vi "Auto Generate Reports.vi"(9 "Report Parameters":T2(array[cluster])=[{"output file suffix"="TSM_SSC", "dir filter"="^\\b(?:(?!SSC|Single SSC)\\w)+\\b"}, {"output file suffix"="SSC", "dir filter"="^SSC|^Single SSC "}], 10 "output file path":path=path "docs", 11 "search dir":path=path "C:/ADIBitbucket/nists19.0_templateproject/Code Modules/Common/Instrument Control") -> (0 "error out":errorcluster={"status"=TRUE, "code"=118, "source"="Invoke Node in VI Documenation MD Report Gen.lvlib:Format VI Information.vi:2500001->VI Documenation MD Report Gen.lvlib:Generate Documentation from VIs.vi->VI Documenation MD Report Gen.lvlib:Auto Generate Reports.vi\n<APPEND>\nMethod Name: <b>Print:VI To HTML</b>"}, 1 "Report Text":string[](array[string]), 3 "Report Files":path[](array[path])=[path "C:/Users/marobert/Desktop/STSDevToolsDocProj/LV Documenation to MD/VI Documenation MD Report Gen/docs/Waveform Acquisition_TSM_SSC.md", path "C:/Users/marobert/Desktop/STSDevToolsDocProj/LV Documenation to MD/VI Documenation MD Report Gen/docs/Waveform Acquisition_SSC.md"])   [LabVIEW 2019, in "MD Generator.lvlib"]
uses:
  MD Generator.lvlib
  subVIs/Filter.ctl
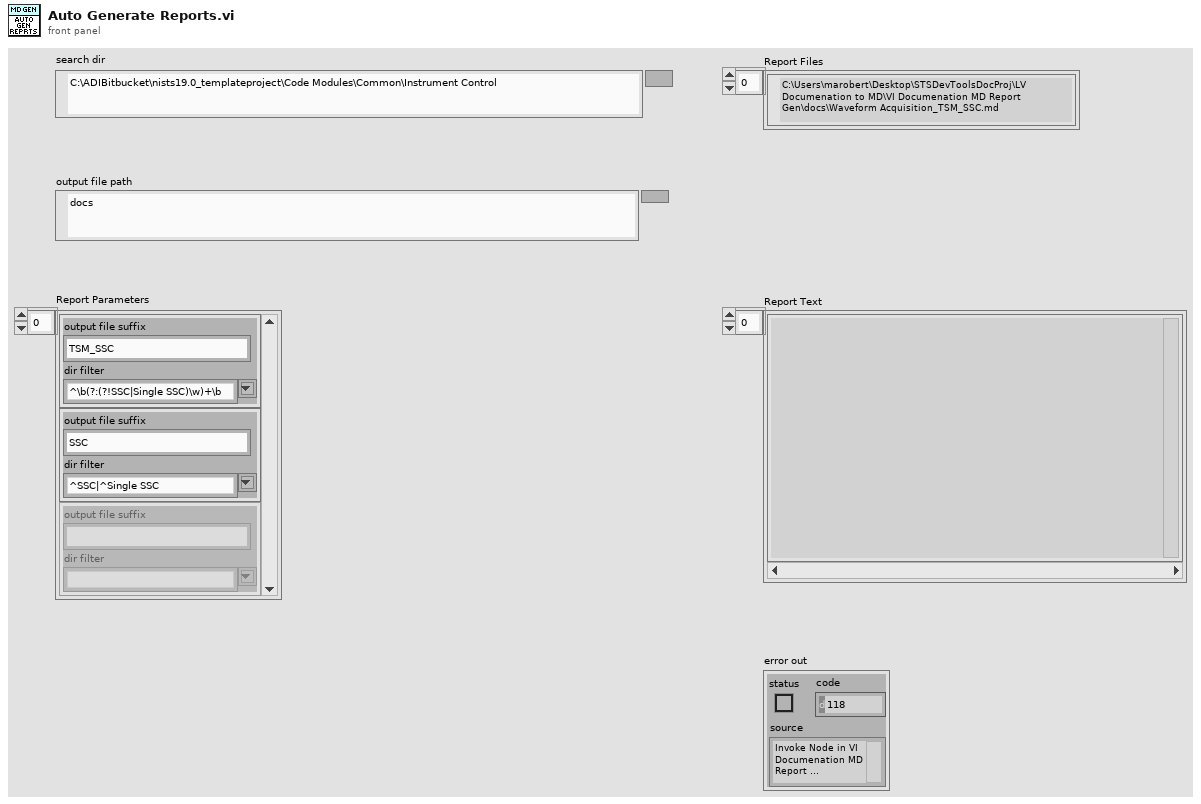
[diagram p1: front panel]
types:
  T1 = typedef "MD Generator.lvlib/Filter.ctl" = string
  T2 = cluster{"output file suffix":string, "dir filter":T1}[]
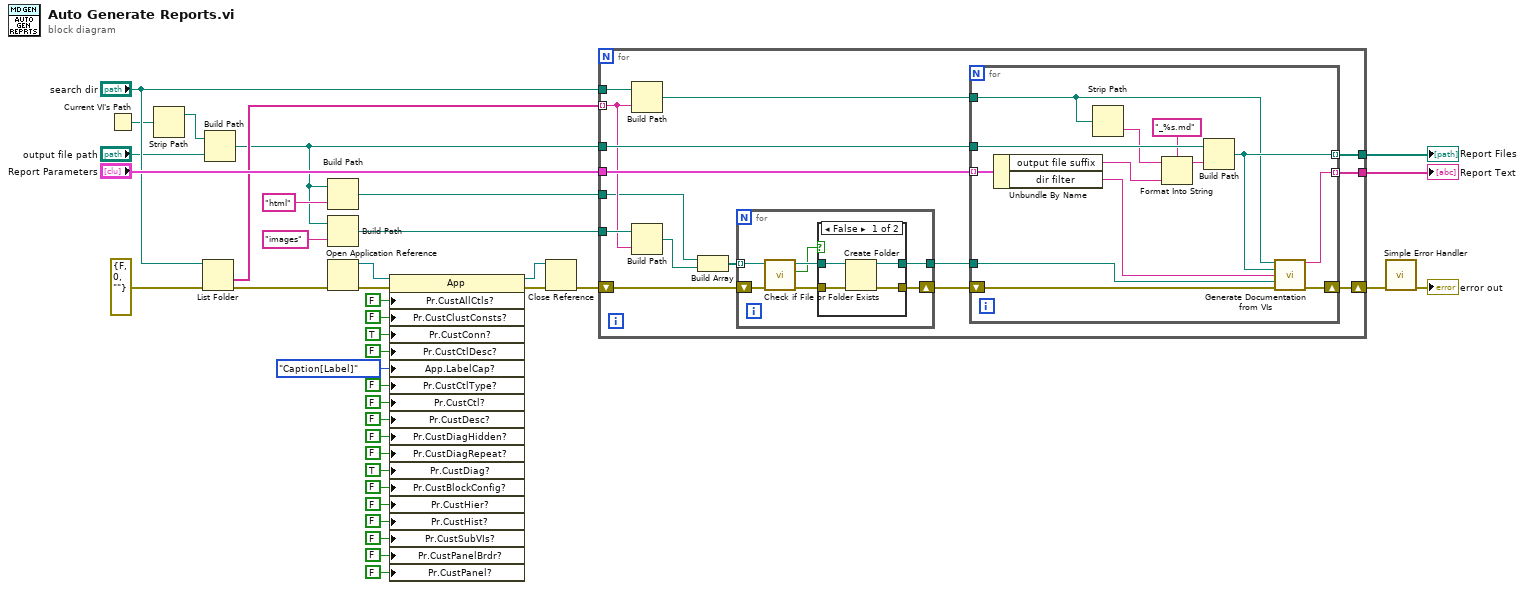
[diagram p0: block diagram]
diagram:
  n1 = Current VI's Path() -> (path=w5:path)
  n2 = Strip Path(path=w5) -> (stripped path=w4:path)  [unwired: 1 out]
  n3 = List Folder(path="search dir", error in=errorcluster {"status"=FALSE, "code"=0, "source"=""} ("error out")) -> (folder names=w33:string[], error out=w10:errorcluster)  [unwired: 2 in, 2 out]
  n4 = Build Path(base path=w4, name or relative path="output file path") -> (appended path=w2:path)
  n5 = Build Path(base path=w2, name or relative path="html") -> (appended path=w1:path)
  n6 = Build Path(base path=w2, name or relative path="images") -> (appended path=w31:path)
  n7 = Open Application Reference(8:w10) -> (0:w29:errorcluster, 3:w8:refnum<vi>)  [unwired: 3 in]
  n8 = property class="App"(reference=w8, error in=w29, "Pr.CustAllCtls?"=FALSE ("Printing:Custom All Controls?"), "Pr.CustClustConsts?"=FALSE ("Printing:Custom Cluster Constants?"), "Pr.CustConn?"=TRUE ("Printing:Custom Connector?"), "Pr.CustCtlDesc?"=FALSE ("Printing:Custom Control Descriptions?"), "App.LabelCap?"=enum16{"Label", "Caption", "Caption[Label]"}."Caption[Label]" ("Printing:Custom Control Label/Caption?"), "Pr.CustCtlType?"=FALSE ("Printing:Custom Control Types?"), "Pr.CustCtl?"=FALSE ("Printing:Custom Controls?"), "Pr.CustDesc?"=FALSE ("Printing:Custom Description?"), "Pr.CustDiagHidden?"=FALSE ("Printing:Custom Diagram Hidden?"), "Pr.CustDiagRepeat?"=FALSE ("Printing:Custom Diagram Repeat?"), "Pr.CustDiag?"=TRUE ("Printing:Custom Diagram?"), "Pr.CustBlockConfig?"=FALSE ("Printing:Custom Express VI Configuration?"), "Pr.CustHier?"=FALSE ("Printing:Custom Hierarchy?"), "Pr.CustHist?"=FALSE ("Printing:Custom History?"), "Pr.CustSubVIs?"=FALSE ("Printing:Custom List of SubVIs?"), "Pr.CustPanelBrdr?"=FALSE ("Printing:Custom Panel Border?"), "Pr.CustPanel?"=FALSE ("Printing:Custom Panel?")) -> (reference out=w7:refnum<vi>, error out=w28:errorcluster)
  n9 = Close Reference(reference=w7, error in (no error)=w28) -> (error out=w9:errorcluster)
  n10 = for {
    tunnel: [w53] -> w37
    tunnel: "search dir" -> [w49]
    tunnel: w31 -> [w46]
    tunnel: "Report Parameters" -> [w52]
    tunnel: w2 -> [w47]
    tunnel: [w50] -> w34
    shift-right: [w54] -> w39
    shift-left: w9 -> [w51]
    tunnel: w33 -> [w45] mode=indexing
    tunnel: w1 -> [w40]
    n11 = Build Path(base path=w49, name or relative path=w45) -> (appended path=w48:path)
    n12 = Build Path(base path=w46, name or relative path=w45) -> (appended path=w42:path)
    n13 = Build Array(w40, w42) -> (w41:path[])
    n14 = for {
      shift-right: [w58] -> w44
      shift-left: w51 -> [w61]
      tunnel: w41 -> [w59] mode=indexing
      tunnel: [w57] -> w43
      n15 = call <vilib>:"Check if File or Folder Exists.vi"("error in (no error)"=w61, "path"=w59) -> ("error out"=w60:errorcluster, "file or folder exists?"=w55:bool, "dup path"=w56:path)  [unwired: 7 in]
      n16 = case shown="False" w55 {
        tunnel: w60 -> [w65 w67]
        tunnel: [w64 w67] -> w58
        tunnel: [w63 w66] -> w57
        tunnel: w56 -> [w62 w66]
        frame False {
          n17 = Create Folder(path (use dialog)=w62, error in=w65) -> (created path=w63:path, error out=w64:errorcluster)  [unwired: 1 in, 1 out]
        }
        frame True {
        }
      }
    }
    n18 = for {
      shift-right: [w80] -> w54
      shift-left: w44 -> [w79]
      tunnel: [w78] -> w53 mode=indexing
      tunnel: w48 -> [w72]
      tunnel: w43 -> [w77]
      tunnel: w52 -> [w76] mode=indexing
      tunnel: w47 -> [w74]
      tunnel: [w73] -> w50 mode=indexing
      n19 = Unbundle By Name(w76) -> ("output file suffix"=w68:string, "dir filter"=w75:T1)
      n20 = Strip Path(path=w72) -> (name=w69:string)  [unwired: 1 out]
      n21 = Format Into String(format string="_%s.md", initial string=w69, w68) -> (resulting string=w71:string)  [unwired: 1 in, 1 out]
      n22 = Build Path(base path=w74, name or relative path=w71) -> (appended path=w73:path)
      n23 = call "Generate Documentation from VIs.vi"("search dir"=w72, "output file path"=w73, "dir filter"=w75, "image dir"=w77, "error in"=w79) -> ("Report"=w78:string, "error out"=w80:errorcluster)  [unwired: 7 in, 2 out]
    }
  }
  "Report Text" <- w37
  "Report Files" <- w34
  n24 = call <vilib>:"Simple Error Handler.vi"("error in (no error)"=w39) -> ("error out"=→"error out":errorcluster)  [unwired: 4 in, 4 out]
